vi "libssh2_sftp_unlink_ex.vi"(8 "error in (no error)":errorcluster, 10 "file":string, 11 "sftp":T1) -> (0 "error out":errorcluster)   [LabVIEW 2017, in "libssh2.lvlib"]
doc: "Delete a file."
uses:
  libssh2.lvlib
  SFTP Refnum.ctl
  Acquire Session.vi
  Release Session.vi
  Not An SFTP Refnum.vi
  <vilib>/Utility/error.llb/Error Cluster From Error Code.vi
  Global Settings.vi
  Read SFTP Refnum.vi
  Read Session Refnum.vi
  <vilib>/Utility/semaphor.llb/Acquire Semaphore.vi
  <vilib>/Utility/semaphor.llb/Release Semaphore.vi
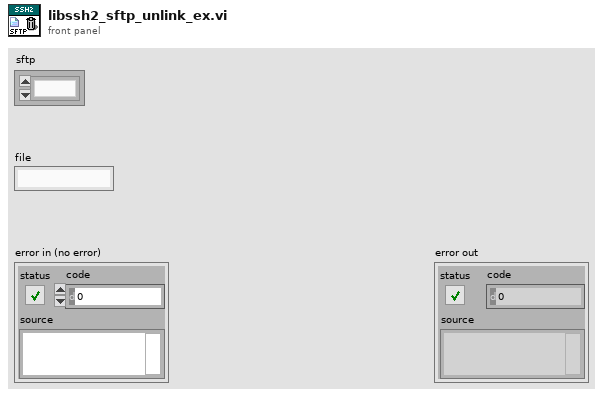
[diagram p1: front panel]
types:
  T1 = typedef "libssh2.lvlib/SFTP Refnum.ctl" = refnum<k1>
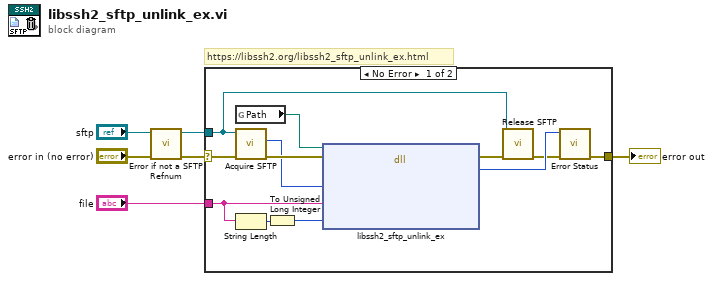
[diagram p0: block diagram]
diagram:
  # "https://libssh2.org/libssh2_sftp_unlink_ex.html"
  n1 = call "Error if not a SFTP Refnum.vi"("error in (no error)"="error in (no error)", "sftp"="sftp") -> ("error out"=w5:errorcluster, "sftp out"=w4:T1)  [unwired: 8 in]
  n2 = case shown="No Error" w5 {
    selector: w5 -> [w17 w19]
    tunnel: w4 -> [w7 _]
    tunnel: [w13 w19] -> w3
    tunnel: "file" -> [w11 _]
    frame No Error {
      n3 = global read "Global Settings.vi" "Path"() -> (w18:path)
      n4 = call "Acquire SFTP.vi"("error in (no error)"=w17, "sftp"=w7) -> ("error out"=w16:errorcluster, "LIBSSH2_SFTP*"=w15:u64)  [unwired: 8 in]
      n5 = String Length(string=w11) -> (length=w10:i32)
      n6 = To Unsigned Long Integer(number=w10) -> (unsigned 32bit integer=w9:u32)
      n7 = dll-call lib="?" fn="libssh2_sftp_unlink_ex"(path in=w18, error in=w16, "sftp"=w15, "filename"=w11, "filename_len"=w9) -> (error out=w14:errorcluster, "return value"=w12:i32)  [unwired: 4 in, 1 out]
      n8 = call "Release SFTP.vi"("error in (no error)"=w14, "sftp"=w7) -> ("error out"=w8:errorcluster)  [unwired: 9 in]
      n9 = call "Error Status.vi"("error in (no error)"=w8, "return value"=w12) -> ("error out"=w13:errorcluster)  [unwired: 8 in, 1 out]
    }
    frame Error {
    }
  }
  "error out" <- w3
